vi "Datasheet SW Calibration File Channel Data.vi"(1 "Channel Data":T1[](array[typedef])) -> (0 "Formatted Channel Values":string[][](array[string]))   [LabVIEW 2011]
uses:
  TDMS/TDMS Channel (Sxx).ctl
  OpenG.LIB/array/array.llb/Filter 1D Array (String)__ogtk.vi
  OpenG.LIB/array/array.llb/Index 1D Array Elements (Variant)__ogtk.vi
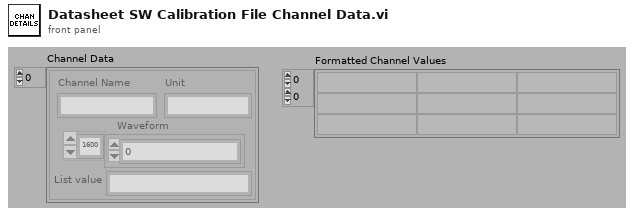
[diagram p1: front panel]
types:
  T1 = typedef "TDMS Channel (Sxx).ctl" = cluster{"Channel Name":string, "Waveform":dbl[], "Unit":string, "List value":string}
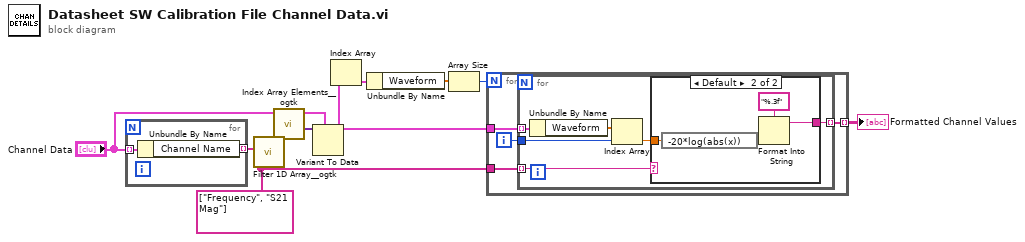
[diagram p0: block diagram]
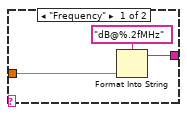
[diagram p2: hidden frame]
diagram:
  w2 = string[] ["Frequency", "S21 Mag"]
  n1 = for {
    tunnel: [w12] -> w7 mode=indexing
    tunnel: "Channel Data" -> [w11] mode=indexing
    n2 = Unbundle By Name(w11) -> ("Channel Name"=w12:string)
  }
  n3 = call-poly "Filter 1D Array__ogtk.vi"("items to filter"=w2, "array"=w7) -> ("filtered item indices"=w6:i32[])  [unwired: 4 in, 1 out]
  n4 = call-poly "Index Array Elements__ogtk.vi"("indices"=w6, "array"="Channel Data") -> ("elements"=w5:variant[])  [unwired: 9 in]
  n5 = Variant To Data(type="Channel Data", Variant=w5) -> (data=w4:T1[])  [unwired: 1 in, 1 out]
  n6 = Index Array(array=w4) -> (element=w10:T1)  [unwired: 1 in]
  n7 = Unbundle By Name(w10) -> ("Waveform"=w9:dbl[])
  n8 = Array Size(array=w9) -> (size(s)=w8:i32)
  n9 = for {
    N: w8 -> [_]
    tunnel: w4 -> [w16]
    tunnel: w2 -> [w14]
    tunnel: [w13] -> w1 mode=indexing
    i -> [w15]
    n10 = for {
      tunnel: w16 -> [w19] mode=indexing
      tunnel: w15 -> [w22]
      tunnel: [w21] -> w13 mode=indexing
      tunnel: w14 -> [w17] mode=indexing
      n11 = Unbundle By Name(w19) -> ("Waveform"=w20:dbl[])
      n12 = Index Array(array=w20, index=w22) -> (element=w18:dbl)
      n13 = case shown="Default" w17 {
        tunnel: [w25 w29] -> w21
        tunnel: w18 -> [w23 w27]
        frame "Frequency" {
          n14 = Format Into String(format string="dB@%.2fMHz", w23) -> (resulting string=w25:string)  [unwired: 2 in, 1 out]
        }
        frame Default {
          n15 = expression code="-20*log(abs(x))"(w27) -> (w26:dbl)
          n16 = Format Into String(format string="%.3f", w26) -> (resulting string=w29:string)  [unwired: 2 in, 1 out]
        }
      }
    }
  }
  "Formatted Channel Values" <- w1
